vi "Labeling.vi"() -> ()   [LabVIEW 2020]
uses:
  Global Variables/Global_Rating.vi
panel:
  out "TEH WANTED POINT":dbl format="%#_13g"
  in  "STOP":bool
  out "Array":T1(array[cluster])
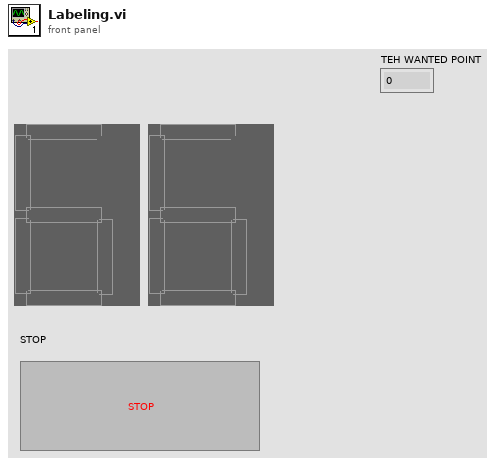
[diagram p1: front panel]
types:
  T1 = cluster{"Boolean":bool, "Boolean 2":bool, "Boolean 3":bool, "Boolean 4":bool, "Boolean 5":bool, "Boolean 6":bool, "Boolean 7":bool}[]
  T2 = cluster{"t[0]":bool, "t[1]":bool, "t[2]":bool, "t[3]":bool, "t[4]":bool, "t[5]":bool, "t[6]":bool}
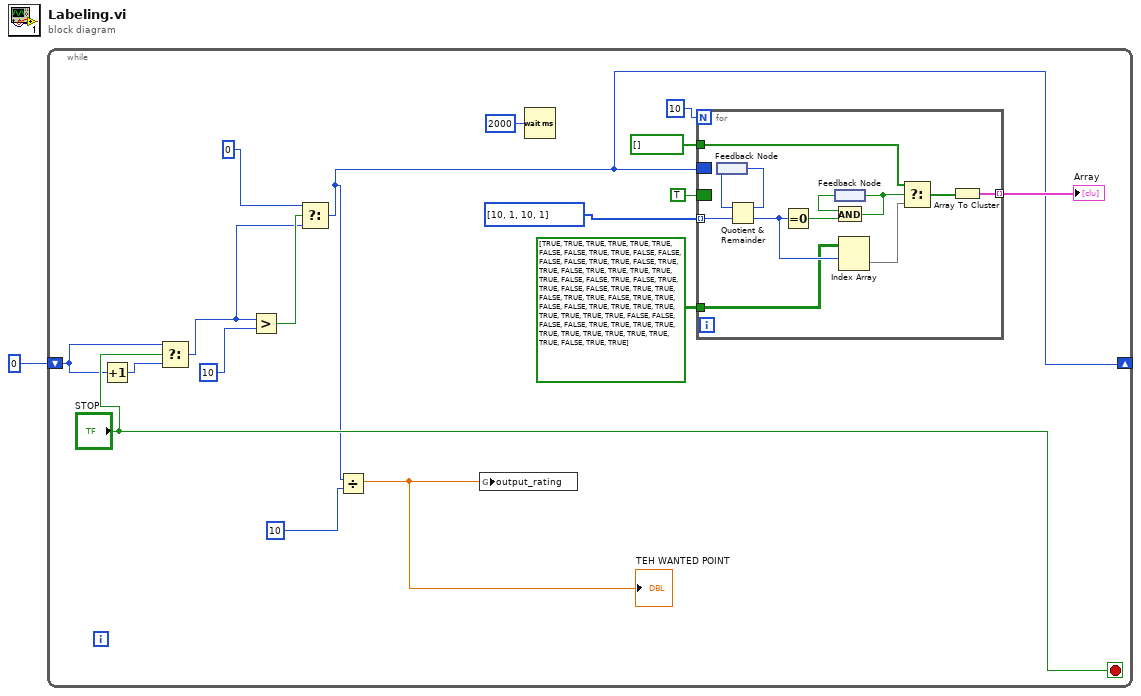
[diagram p0: block diagram]
diagram:
  n1 = while {
    shift-right: [w6] -> _
    shift-left: 0 -> [w5]
    stop <- "STOP" stop-if-true
    n2 = Increment(x=w5) -> (x+1=w4:i32)
    n3 = Select(t=w5, s="STOP", f=w4) -> (s? t:f=w3:i32)
    n4 = Greater?(x=w3, y=10) -> (0:w8:bool)
    n5 = Select(t=0, s=w8, f=w3) -> (s? t:f=w6:i32)
    n6 = Divide(x=w6, y=10) -> (x/y=w11:dbl)
    "TEH WANTED POINT" <- w11
    n7 = global write "Global_Rating.vi" "output_rating"(w11) -> ()
    n8 = Wait (ms)(milliseconds to wait=u32 2000) -> ()  [unwired: 1 out]
    n9 = for {
      N: 10 -> [_]
      border: w6 -> [_]
      tunnel: i32[] [10, 1, 10, 1] -> [w28] mode=indexing
      tunnel: [w27] -> w18 mode=indexing
      border: TRUE -> [_]
      tunnel: bool[][] [[TRUE, TRUE, TRUE, TRUE, TRUE, TRUE, FALSE], [FALSE, TRUE, TRUE, FALSE, FALSE, FALSE, FALSE], [TRUE, TRUE, FALSE, TRUE, TRUE, FALSE, TRUE], [TRUE, TRUE, TRUE, TRUE, FALSE, FALSE, TRUE], [FALSE, TRUE, TRUE, FALSE, FALSE, TRUE, TRUE], [TRUE, FALSE, TRUE, TRUE, FALSE, TRUE, TRUE], [FALSE, FALSE, TRUE, TRUE, TRUE, TRUE, TRUE], [TRUE, TRUE, TRUE, FALSE, FALSE, FALSE, FALSE], [TRUE, TRUE, TRUE, TRUE, TRUE, TRUE, TRUE], [TRUE, TRUE, TRUE, TRUE, FALSE, TRUE, TRUE]] -> [w20]
      tunnel: bool[] [] ("t") -> [w19]
      n10 = feedback #1() -> (w29:i32)
      n11 = Quotient & Remainder(x=w29, y=w28) -> (x-y*floor(x/y)=w30:i32, floor(x/y)=w26:i32)
      n12 = feedback-in #1(w30) -> ()
      n13 = Equal To 0?(x=w26) -> (x = 0?=w25:bool)
      n14 = feedback #2() -> (w24:bool)
      n15 = And(x=w24, y=w25) -> (x .and. y?=w21:bool)
      n16 = feedback-in #2(w21) -> ()
      n17 = Index Array(array=w20, index (row)=w26) -> (element=w23:bool[])  [unwired: 1 in]
      n18 = Select(t=w19, s=w21, f=w23) -> (s? t:f=w22:bool[])
      n19 = Array To Cluster(array=w22) -> (cluster=w27:T2)
    }
    "Array" <- w18
  }
